vi "TestDataTypes.vi"() -> ()   [LabVIEW 2018]
uses:
  e940efb5-caef-4995-b771-34a9a67a4301.vi
  a1c0f9d2-26ec-4268-8f6b-11632fd035ce.vi
  f188b178-77fc-44d9-88fc-7297ac981d4f.vi
  dee43fe5-3f2e-4d55-bcb5-f2ae15acc2d8.vi
  23cfde3f-9cb4-4cf9-8fcd-1987ade9aab5.vi
  b3c14a34-2208-4527-8448-13172d94b60f.vi
  e940efb5-caef-4995-b771-34a9a67a4301.vi/da2973d5-6e52-4aa2-ba25-03978c79fba6.vi
  a1c0f9d2-26ec-4268-8f6b-11632fd035ce.vi/bddab56b-1449-42f4-8f39-79192b4a8e38.vi
  f188b178-77fc-44d9-88fc-7297ac981d4f.vi/ab090b8d-f029-4e83-b2bc-2de9c8910127.vi
  dee43fe5-3f2e-4d55-bcb5-f2ae15acc2d8.vi/f891aedf-ed6c-4848-a557-8a098f1dd0ec.vi
  23cfde3f-9cb4-4cf9-8fcd-1987ade9aab5.vi/899041e1-1145-4b2a-9748-2bfcb047d807.vi
  b3c14a34-2208-4527-8448-13172d94b60f.vi/179fd6aa-71b3-496e-84b5-5de811675b58.vi
  feGEM DataPacker.lvlib
panel:
  in  "MIDAS Server":string="my_midas_server.domain"
  in  "MIDAS Sever Port":u16=12345
  out "log bool error out":errorcluster
  in  "bool array":bool[](array[boolean])
  out "log int16_t error out":errorcluster
  in  "uint16_t array":u16[](array[numeric])=[0, 0, 0, 0, 0, 1, 1, 1, 1, 1]
  out "log int32_t error out":errorcluster
  in  "int32_t array":i32[](array[numeric])=[0, 0, 0, 0, 0, 1, 1, 1, 1, 1]
  out "log uint32_t error out":errorcluster
  in  "uint32_t array":u32[](array[numeric])=[0, 0, 0, 0, 0, 1, 1, 1, 1, 1]
  in  "Single (float) array":sgl[](array[numeric])=[0.1, 0.2, 0.3, 0.4, 0.5, 0.6, 0.7, 0.8, 0.9, 1.0]
  out "log float error out":errorcluster
  out "Announcement Error":errorcluster
  in  "stop":bool
  out "Log doubles error out":errorcluster
  in  "Double array":dbl[](array[numeric])=[0.1, 0.2, 0.3, 0.4, 0.5, 0.6, 0.7, 0.8, 0.9, 1.0]
  out "Get Run Status Error out":errorcluster
  out "Run Status":string
  out "Get RunNumber Error out":errorcluster
  out "RUNNO":i32
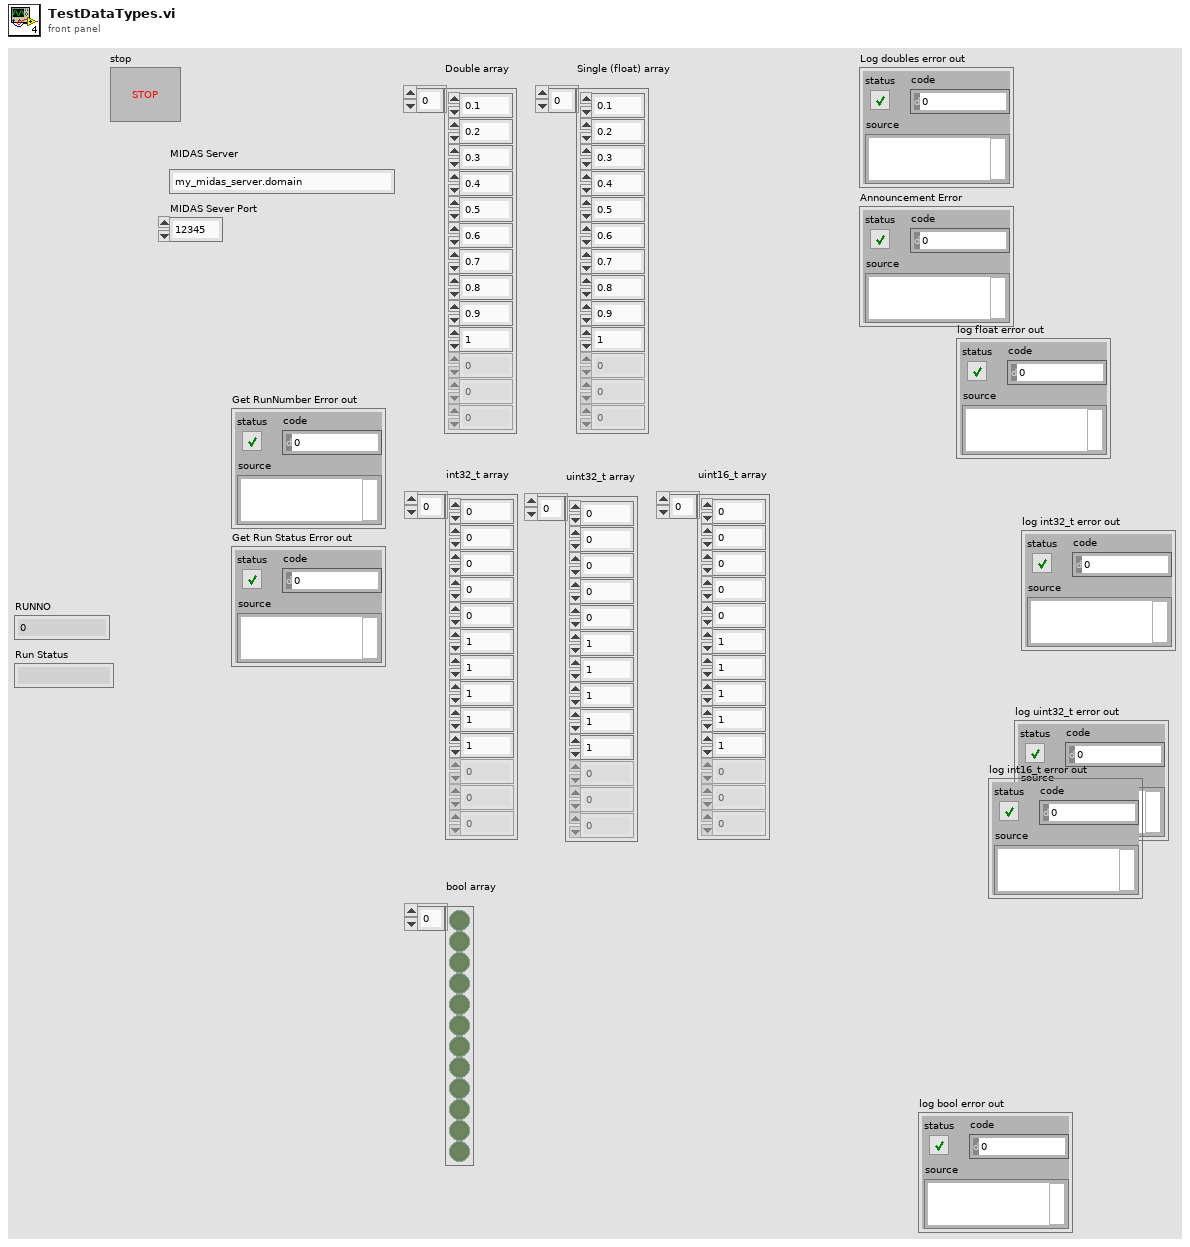
[diagram p1: front panel]
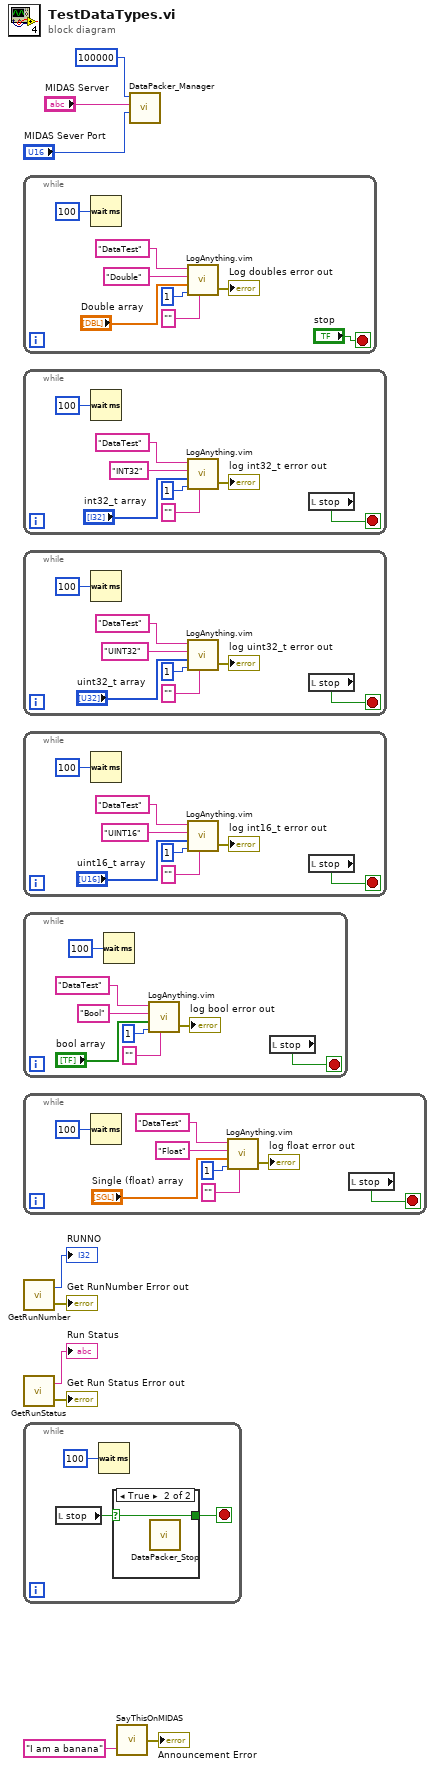
[diagram p0: block diagram]
diagram:
  n1 = while {
    stop <- "stop" stop-if-true
    n2 = Wait (ms)(milliseconds to wait=u32 100) -> ()  [unwired: 1 out]
    n3 = call "LogAnything.vim"("Equipment description"="", "Period to update history plots (seconds)\nUnset (65535) = Use MIDAS default in ODB\n0 = Record but do not put in histories"=1 ("Rate to update history plots"), "Array"="Double array", "Var Name"="Double", "Category"="DataTest") -> ("error out"=→"Log doubles error out":errorcluster)  [unwired: 2 in]
  }
  n4 = while {
    stop <- w18 stop-if-true
    n5 = Wait (ms)(milliseconds to wait=u32 100) -> ()  [unwired: 1 out]
    n6 = call "LogAnything.vim"("Equipment description"="", "Period to update history plots (seconds)\nUnset (65535) = Use MIDAS default in ODB\n0 = Record but do not put in histories"=1 ("Rate to update history plots"), "Array"="int32_t array", "Var Name"="INT32", "Category"="DataTest") -> ("error out"=→"log int32_t error out":errorcluster)  [unwired: 2 in]
    n7 = local read "stop"() -> (w18:bool)
  }
  n8 = while {
    stop <- w26 stop-if-true
    n9 = Wait (ms)(milliseconds to wait=u32 100) -> ()  [unwired: 1 out]
    n10 = call "LogAnything.vim"("Equipment description"="", "Period to update history plots (seconds)\nUnset (65535) = Use MIDAS default in ODB\n0 = Record but do not put in histories"=1 ("Rate to update history plots"), "Array"="uint32_t array", "Var Name"="UINT32", "Category"="DataTest") -> ("error out"=→"log uint32_t error out":errorcluster)  [unwired: 2 in]
    n11 = local read "stop"() -> (w26:bool)
  }
  n12 = while {
    stop <- w34 stop-if-true
    n13 = Wait (ms)(milliseconds to wait=u32 100) -> ()  [unwired: 1 out]
    n14 = call "LogAnything.vim"("Equipment description"="", "Period to update history plots (seconds)\nUnset (65535) = Use MIDAS default in ODB\n0 = Record but do not put in histories"=1 ("Rate to update history plots"), "Array"="uint16_t array", "Var Name"="UINT16", "Category"="DataTest") -> ("error out"=→"log int16_t error out":errorcluster)  [unwired: 2 in]
    n15 = local read "stop"() -> (w34:bool)
  }
  n16 = while {
    stop <- w42 stop-if-true
    n17 = Wait (ms)(milliseconds to wait=u32 100) -> ()  [unwired: 1 out]
    n18 = call "LogAnything.vim"("Equipment description"="", "Period to update history plots (seconds)\nUnset (65535) = Use MIDAS default in ODB\n0 = Record but do not put in histories"=1 ("Rate to update history plots"), "Array"="bool array", "Var Name"="Bool", "Category"="DataTest") -> ("error out"=→"log bool error out":errorcluster)  [unwired: 2 in]
    n19 = local read "stop"() -> (w42:bool)
  }
  n20 = while {
    stop <- w50 stop-if-true
    n21 = Wait (ms)(milliseconds to wait=u32 100) -> ()  [unwired: 1 out]
    n22 = call "LogAnything.vim"("Equipment description"="", "Period to update history plots (seconds)\nUnset (65535) = Use MIDAS default in ODB\n0 = Record but do not put in histories"=1 ("Rate to update history plots"), "Array"="Single (float) array", "Var Name"="Float", "Category"="DataTest") -> ("error out"=→"log float error out":errorcluster)  [unwired: 2 in]
    n23 = local read "stop"() -> (w50:bool)
  }
  n24 = call "GetRunNumber.vi"() -> ("error out"=→"Get RunNumber Error out":errorcluster, "RunNumber"=→"RUNNO":i32)  [unwired: 2 in]
  n25 = call "GetRunStatus.vi"() -> ("error out"=→"Get Run Status Error out":errorcluster, "Run Status"=→"Run Status":string)  [unwired: 2 in]
  n26 = while {
    stop <- w59 stop-if-true
    n27 = local read "stop"() -> (w58:bool)
    n28 = Wait (ms)(milliseconds to wait=u32 100) -> ()  [unwired: 1 out]
    n29 = case shown="True" w58 {
      selector: w58 -> [w61 w62]
      tunnel: [w61 w62] -> w59
      frame False {
      }
      frame True {
        n30 = call "DataPacker_Stop.vi"() -> ()  [unwired: 12 in]
      }
    }
  }
  n31 = call "SayThisOnMIDAS.vi"("String"="I am a banana") -> ("error out"=→"Announcement Error":errorcluster)  [unwired: 1 in]
  n32 = call "DataPacker_Manager.vi"("MIDAS Sever Port"="MIDAS Sever Port", "MIDAS Server"="MIDAS Server", "Override Max Event size (Data rate bytes/s). Use MIDAS Default = 0"=u32 100000 ("Override Max Event size (Data rate kb/s). Use MIDAS Default = 0")) -> ()  [unwired: 9 in]
